vi "DoOperationStaticDispatchMethod Wrapper - Reentrant.vi"(8 "error in (no error)":errorcluster, 11 "SimpleArithmetic in":refnum<class "SimpleArithmetic - Reentrant.lvclass">) -> (0 "error out":errorcluster, 3 "SimpleArithmetic out":refnum<class "SimpleArithmetic - Reentrant.lvclass">)   [LabVIEW 2013]
uses:
  SimpleArithmetic - Reentrant.lvclass
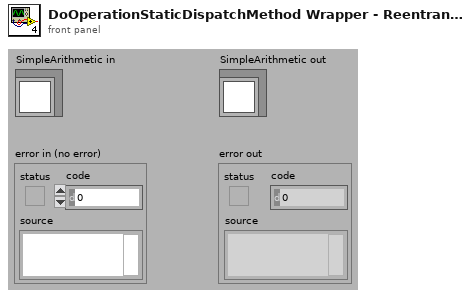
[diagram p1: front panel]
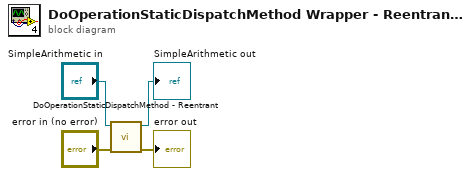
[diagram p0: block diagram]
diagram:
  n1 = call "DoOperationStaticDispatchMethod - Reentrant.vi"("error in (no error)"="error in (no error)", "SimpleArithmetic in"="SimpleArithmetic in") -> ("error out"=→"error out":errorcluster, "SimpleArithmetic out"=→"SimpleArithmetic out":refnum<class "SimpleArithmetic - Reentrant.lvclass">)  [unwired: 8 in]
